vi "SVT Spectrum Peak Search.vi"   [LabVIEW 2017]
doc: "Performs a peak search on a spectrum or spectra in the frequency domain. Detects single or multiple peaks in Power, PSD, COP, and FFT [Mag] spectra. You can use this polymorphic VI to analyze a single spectrum or N spectra. The data type you wire to the <B>spectrum</B> input determines the polymorphic instance to use."
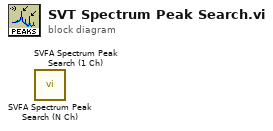
[diagram p0: block diagram]
diagram:
  n1 = call <vilib>:"SVFA Spectrum Peak Search (N Ch).vi"() -> ()  [unwired: 15 in, 5 out]
  n2 = call <vilib>:"SVFA Spectrum Peak Search (1 Ch).vi"() -> ()  [unwired: 15 in, 5 out]
